vi "FVIR_LDO_Oil_Machine.vi"(8 "error in":errorcluster, 11 "Message Queues":T1) -> (0 "error out":errorcluster)   [LabVIEW 2020]
uses:
  Message Queue/All Message Queues.ctl
  Message Queue/Message Cluster.ctl
  Drivers/Unist Quantum/Type Definitions/UNIST Fluid Rate.ctl
  Message Queue/Enqueue Message (Single).vi
  Message Queue/Message Queue.lvlib
panel:
  out "Loop Count":i32
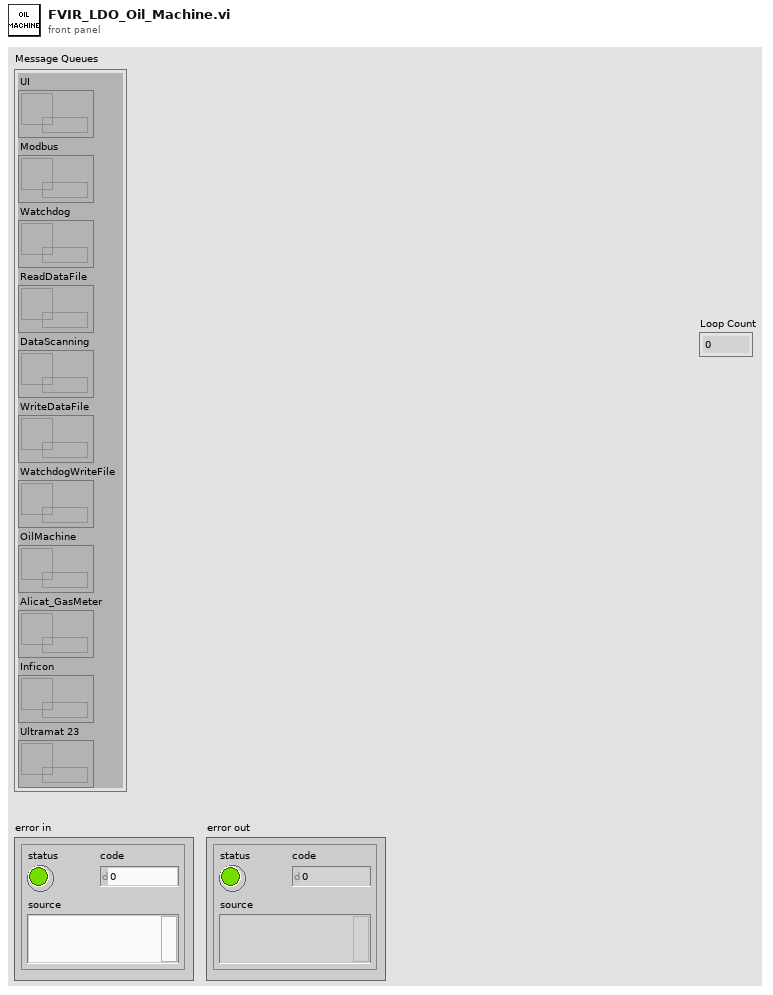
[diagram p1: front panel]
types:
  T1 = typedef "Message Queue.lvlib/All Message Queues.ctl" = cluster{"UI":refnum<queue>, "Modbus":refnum<queue>, "Watchdog":refnum<queue>, "ReadDataFile":refnum<queue>, "DataScanning":refnum<queue>, "WriteDataFile":refnum<queue>, "WatchdogWriteFile":refnum<queue>, "OilMachine":refnum<queue>, "Alicat_GasMeter":refnum<queue>, "Inficon":refnum<queue>, "Ultramat 23":refnum<queue>}
  T2 = typedef "UNIST Fluid Rate.ctl" = string
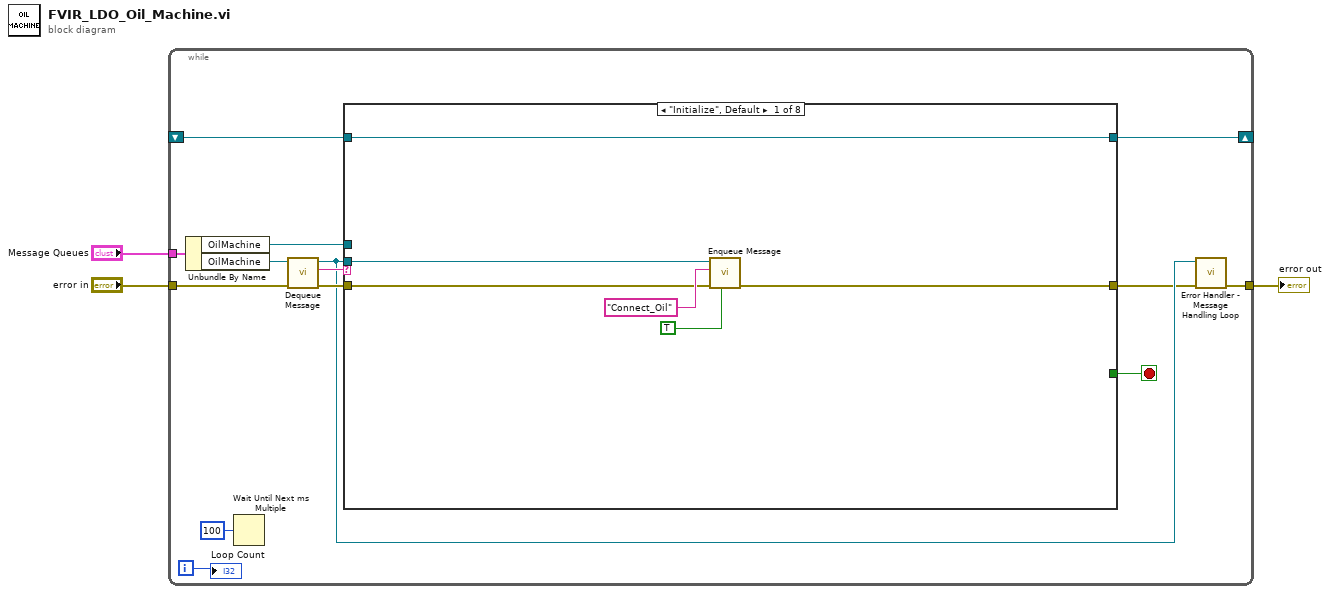
[diagram p0: block diagram]
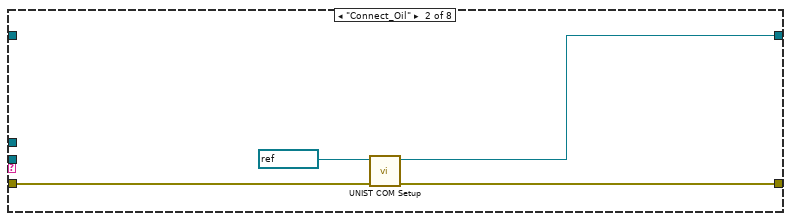
[diagram p2: hidden frame]
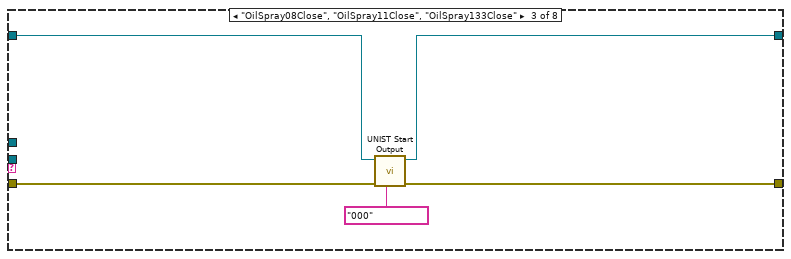
[diagram p3: hidden frame]
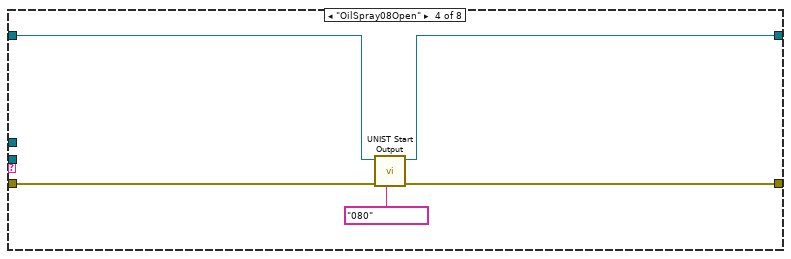
[diagram p4: hidden frame]
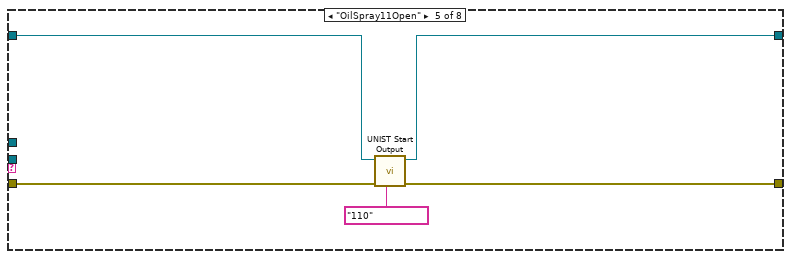
[diagram p5: hidden frame]
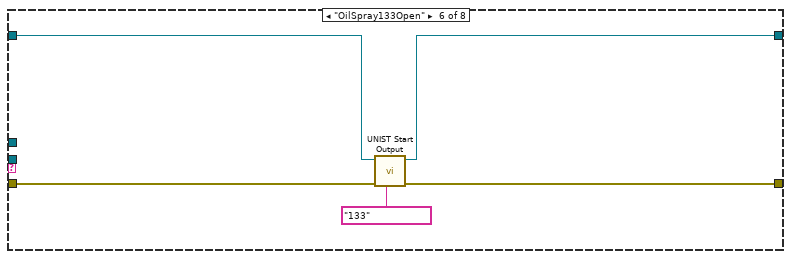
[diagram p6: hidden frame]
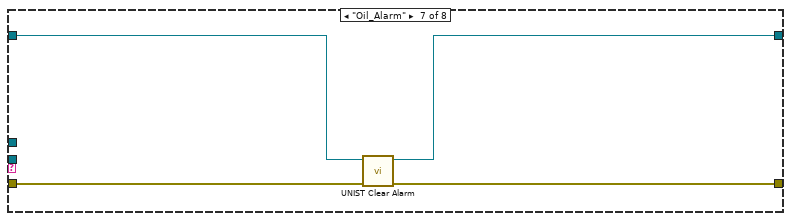
[diagram p7: hidden frame]
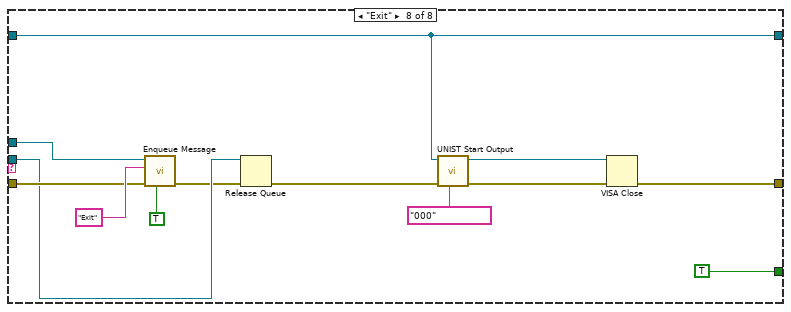
[diagram p8: hidden frame]
diagram:
  n1 = while {
    tunnel: "Message Queues" -> [w17]
    tunnel: "error in" -> [w15]
    tunnel: [w9] -> w1
    shift-right: [w7] -> _
    shift-left: _ -> [w6]
    i -> [w4]
    stop <- w12 stop-if-true
    n2 = Unbundle By Name(w17) -> ("OilMachine"=w11:refnum<queue>, "OilMachine"=w16:refnum<queue>)
    n3 = Wait Until Next ms Multiple(millisecond multiple=u32 100) -> ()  [unwired: 1 out]
    n4 = call "Dequeue Message.vi"("error in (no error)"=w15, "Message Queue"=w16) -> ("error out"=w13:errorcluster, "Message"=w14:string, "dup Message Queue"=w10:refnum<queue>)  [unwired: 6 in, 1 out]
    n5 = case shown="\"Initialize\", Default" w14 {
      tunnel: w13 -> [w21 w27 w32 w37 w42 w47 w51 w60]
      tunnel: [w20 w26 w31 w36 w41 w46 w50 w57] -> w8
      tunnel: [_ _ _ _ _ _ _ TRUE] -> w12
      tunnel: w11 -> [_ _ _ _ _ _ _ w61]
      tunnel: w10 -> [w19 _ _ _ _ _ _ w59]
      tunnel: [w23 w24 w29 w34 w39 w44 w48 w53] -> w7
      tunnel: w6 -> [w23 _ w30 w35 w40 w45 w49 w53]
      frame "Initialize", Default {
        n6 = call-poly "Enqueue Message.vi"("Priority Message? (F)"=TRUE, "error in (no error)"=w21, "Message"="Connect_Oil", "Message Queue"=w19) -> ("error out"=w20:errorcluster)  [unwired: 6 in, 1 out]
      }
      frame "Connect_Oil" {
        n7 = call "UNIST COM Setup.vi"("error in (no error)"=w27, "VISA Refnum in"=refnum<visa-resource-name> "UNIST") -> ("error out"=w26:errorcluster, "VISA Refnum out"=w24:refnum<visa-resource-name>)  [unwired: 8 in]
      }
      frame "OilSpray08Close", "OilSpray11Close", "OilSpray133Close" {
        n8 = call "UNIST Start Output.vi"("Fluid Rate (CC/MIN)"=T2 "000", "error in (no error)"=w32, "VISA Refnum in"=w30) -> ("error out"=w31:errorcluster, "VISA Refnum out"=w29:refnum<visa-resource-name>)  [unwired: 7 in]
      }
      frame "OilSpray08Open" {
        n9 = call "UNIST Start Output.vi"("Fluid Rate (CC/MIN)"=T2 "080", "error in (no error)"=w37, "VISA Refnum in"=w35) -> ("error out"=w36:errorcluster, "VISA Refnum out"=w34:refnum<visa-resource-name>)  [unwired: 7 in]
      }
      frame "OilSpray11Open" {
        n10 = call "UNIST Start Output.vi"("Fluid Rate (CC/MIN)"=T2 "110", "error in (no error)"=w42, "VISA Refnum in"=w40) -> ("error out"=w41:errorcluster, "VISA Refnum out"=w39:refnum<visa-resource-name>)  [unwired: 7 in]
      }
      frame "OilSpray133Open" {
        n11 = call "UNIST Start Output.vi"("Fluid Rate (CC/MIN)"=T2 "133", "error in (no error)"=w47, "VISA Refnum in"=w45) -> ("error out"=w46:errorcluster, "VISA Refnum out"=w44:refnum<visa-resource-name>)  [unwired: 7 in]
      }
      frame "Oil_Alarm" {
        n12 = call "UNIST Clear Alarm.vi"("error in (no error)"=w51, "VISA Refnum in"=w49) -> ("error out"=w50:errorcluster, "VISA Refnum out"=w48:refnum<visa-resource-name>)  [unwired: 8 in]
      }
      frame "Exit" {
        n13 = call-poly "Enqueue Message.vi"("Priority Message? (F)"=TRUE, "error in (no error)"=w60, "Message"="Exit", "Message Queue"=w61) -> ("error out"=w58:errorcluster)  [unwired: 6 in, 1 out]
        n14 = Release Queue(queue=w59, error in (no error)=w58) -> (error out=w55:errorcluster)  [unwired: 1 in, 2 out]
        n15 = call "UNIST Start Output.vi"("Fluid Rate (CC/MIN)"=T2 "000", "error in (no error)"=w55, "VISA Refnum in"=w53) -> ("error out"=w54:errorcluster, "VISA Refnum out"=w52:refnum<visa-resource-name>)  [unwired: 7 in]
        n16 = VISA Close(VISA resource name=w52, error in (no error)=w54) -> (error out=w57:errorcluster)
      }
    }
    n17 = call "Error Handler - Message Handling Loop.vi"("error in (no error)"=w8, "Message Queue"=w10) -> ("dup error in"=w9:errorcluster)  [unwired: 8 in, 1 out]
    "Loop Count" <- w4
  }
  "error out" <- w1
